vi "XIPIN_DSP48_Macro_3_0.vi"   [LabVIEW 2017]
doc: "The Xilinx LogiCORE DSP48 Macro provides an easy to use interface which abstracts the DSP Slice configuration and simplifies its dynamic operation by enabling the specification of multiple operations via a set of user defined arithmetic expressions. The operations are enumerated and can be selected by the user via single port on the generated IP.\n------------------------------------\n<b>Need License</b> : No"
uses:
  <vilib>/rvi/XilinxIP/XIPIN_XNode/niFpgaXIPIN.xnode
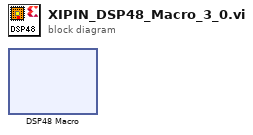
[diagram p0: block diagram]
diagram:
  n1 = xnode ("DSP48 Macro")() -> ()
